vi "Teleop.vi"(10 "Match Info":T2={"Autonomous Elapsed Seconds"=0.0, "TeleOp Elapsed Seconds"=0.0, "Disabled Elapsed Seconds"=0.0, "Visited Autonomous"=FALSE, "Visited TeleOp"=FALSE, "Visited Disabled"=FALSE, "Autonomous Settings"={"Autonomous Style"=enum."Independent", "VI Refnum"=refnum}}, 11 "Call Context":T3) -> ()   [LabVIEW 2014]
doc: "This VI is called for each TeleOp packet received from the DS where the robot is not disabled. It is often used to read from the joysticks and update I/O or to update setpoints for timed control loops. It should complete and return within 20 milliseconds or it may miss DS packets."
uses:
  <vilib>/Rock Robotics/WPI/DriverStation/WPI_DriverStationDerivedRobotMode.ctl
  <vilib>/Rock Robotics/WPI/DriverStation/WPI_DriverStationMatch Info.ctl
  <vilib>/Rock Robotics/WPI/Joystick/WPI_JoystickGetSetRefNum.vi
  Botones Global.vi
  <vilib>/Rock Robotics/Network Tables/SD Write Boolean Array.vi
  <vilib>/Rock Robotics/Network Tables/SD Write Numeric Array.vi
  <vilib>/Rock Robotics/Network Tables/SD Read Boolean.vi
  <vilib>/Rock Robotics/Network Tables/SD Read Number.vi
  Drive Global.vi
  2283_Outputs autonomo.vi
panel:
  in  "Outputs autonomo":T1
  in  "drive":cluster{"Eje 0":dbl, "Eje 1":dbl, "Eje 2":dbl}
  out "Sample Slider 0":dbl(slide) scale=0.0..5.0
  out "Sample Boolean 1":bool
  out "Sample Boolean 0":bool
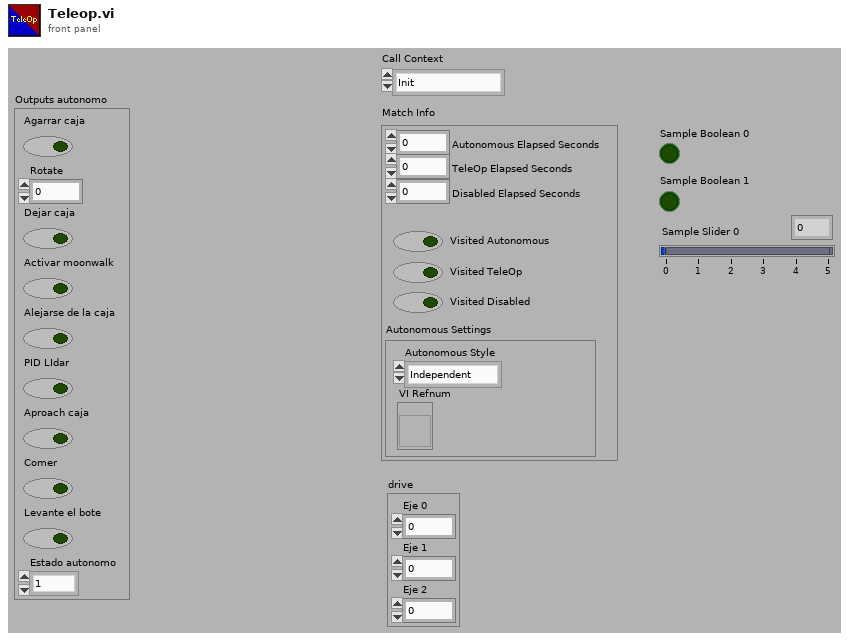
[diagram p1: front panel]
types:
  T1 = cluster{"Agarrar caja":bool, "Rotate":dbl, "Dejar caja":bool, "Activar moonwalk":bool, "Alejarse de la caja":bool, "PID LIdar":bool, "Aproach caja":bool, "Comer":bool, "Levante el bote":bool, "Estado autonomo":enum16{"1", "2", "3", "4", "5", "6", "7", "8", "9", "10", "11", "12"}}
  T2 = typedef "WPI_DriverStationMatch Info.ctl" = cluster{"Autonomous Elapsed Seconds":dbl, "TeleOp Elapsed Seconds":dbl, "Disabled Elapsed Seconds":dbl, "Visited Autonomous":bool, "Visited TeleOp":bool, "Visited Disabled":bool, "Autonomous Settings":cluster{"Autonomous Style":enum16{"Iterative", "Independent"}, "VI Refnum":refnum<vi>}}
  T3 = typedef "WPI_DriverStationDerivedRobotMode.ctl" = enum16{"Init", "Execute", "Stop"}
  T4 = typedef "WPI_JoystickDevRef.ctl" = cluster{"Device":T5}
  T5 = typedef "WPI_JoystickDeviceEnum.ctl" = enum16{"USB 0", "USB 1", "USB 2", "USB 3", "USB 4", "USB 5"}
  T6 = cluster{"Axes[0]":dbl, "Axes[1]":dbl, "Axes[2]":dbl, "Axes[3]":dbl, "Axes[4]":dbl, "Axes[5]":dbl, "Axes[6]":dbl, "Axes[7]":dbl, "Axes[8]":dbl}
  T7 = cluster{"Buttons[0]":bool, "Buttons[1]":bool, "Buttons[2]":bool, "Buttons[3]":bool, "Buttons[4]":bool, "Buttons[5]":bool, "Buttons[6]":bool, "Buttons[7]":bool, "Buttons[8]":bool}
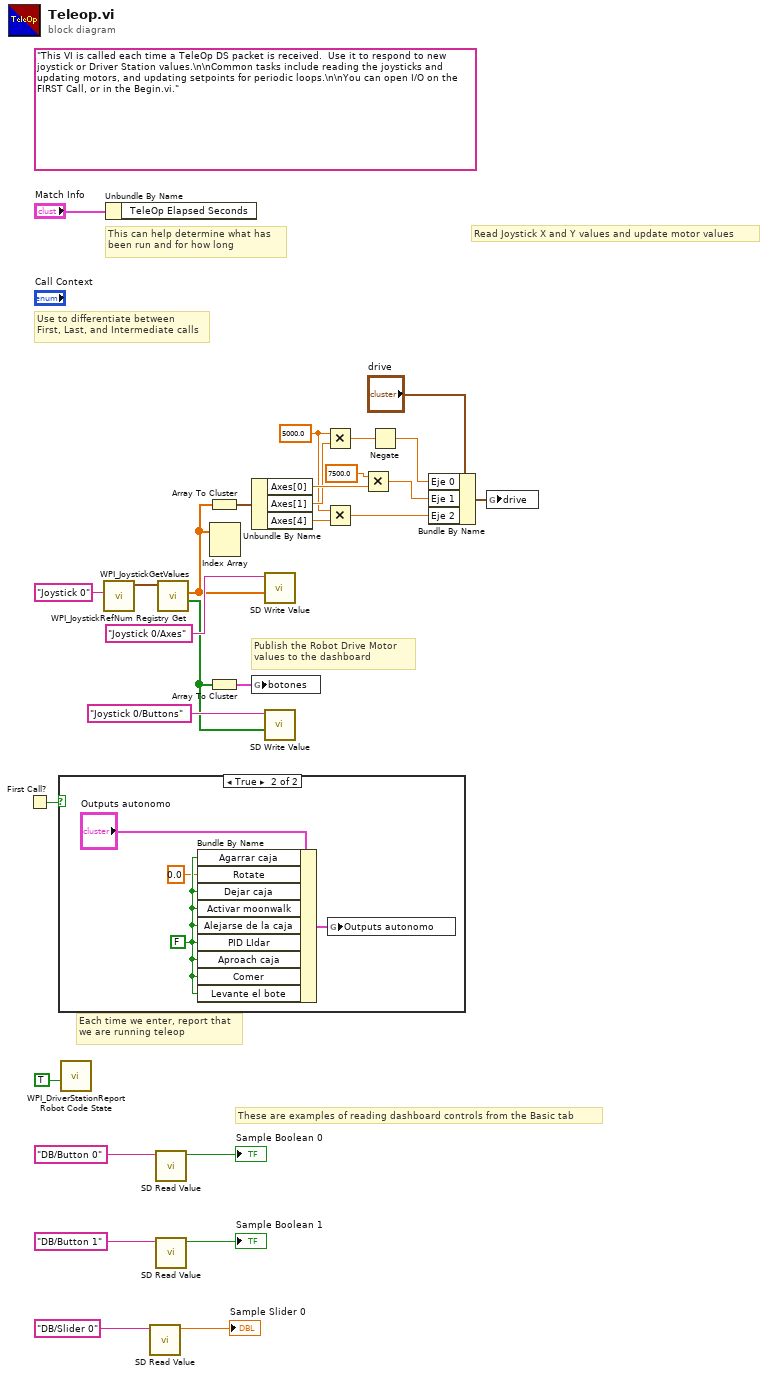
[diagram p0: block diagram]
diagram:
  w6 = 5000.0
  (unwired) "This VI is called each time a TeleOp DS packet is received.  Use it to respond to new joystick or Driver Station values.\n\nCommon tasks include reading the joysticks and updating motors, and updating setpoints for periodic loops.\n\nYou can open I/O on the FIRST Call, or in the Begin.vi."
  # "These are examples of reading dashboard controls from the Basic tab"
  # "Publish the Robot Drive Motor\nvalues to the dashboard"
  # "Each time we enter, report that\nwe are running teleop"
  # "Use to differentiate between\nFirst, Last, and Intermediate calls"
  # "This can help determine what has\nbeen run and for how long"
  # "Read Joystick X and Y values and update motor values"
  n1 = First Call?() -> (First Call?: T/F=w1:bool)
  n2 = case shown="True" w1 {
    frame False {
    }
    frame True {
      w30 = FALSE ("Agarrar caja")
      n3 = Bundle By Name(cluster="Outputs autonomo", "Agarrar caja"=w30, "Rotate"=0.0, "Dejar caja"=w30, "Activar moonwalk"=w30, "Alejarse de la caja"=w30, "PID LIdar"=w30, "Aproach caja"=w30, "Comer"=w30, "Levante el bote"=w30) -> (w32:T1)
      n4 = global write "2283_Outputs autonomo.vi" "Outputs autonomo"(w32) -> ()
    }
  }
  n5 = call <vilib>:"WPI_DriverStationReport Robot Code State.vi"("TeleOp"=TRUE ("Autonomous")) -> ()  [unwired: 10 in, 1 out]
  n6 = call <vilib>:"WPI_JoystickRefNum Registry Get.vi"("refnum name"="Joystick 0") -> ("JoystickDevRef"=w26:T4)  [unwired: 1 in, 9 out]
  n7 = Unbundle By Name("Match Info") -> ()  [unwired: 1 out]
  n8 = call-poly <vilib>:"SD Read Value.vi"("Name"="DB/Slider 0" ("refnum name")) -> ("Numeric"=→"Sample Slider 0":dbl)  [unwired: 8 in, 2 out]
  n9 = call-poly <vilib>:"SD Read Value.vi"("Name"="DB/Button 0" ("refnum name")) -> ("Boolean"=→"Sample Boolean 0":bool)  [unwired: 8 in, 2 out]
  n10 = call-poly <vilib>:"SD Read Value.vi"("Name"="DB/Button 1" ("refnum name")) -> ("Boolean"=→"Sample Boolean 1":bool)  [unwired: 8 in, 2 out]
  n11 = call <vilib>:"WPI_JoystickGetValues.vi"("JoystickDevRef"=w26) -> ("Buttons"=w12:bool[], "Axes"=w16:dbl[])  [unwired: 6 in, 3 out]
  n12 = Array To Cluster(array=w16) -> (cluster=w15:T6)
  n13 = Array To Cluster(array=w12) -> (cluster=w11:T7)
  n14 = Index Array(array=w16) -> ()  [unwired: 2 in, 2 out]
  n15 = Unbundle By Name(w15) -> ("Axes[0]"=w10:dbl, "Axes[1]"=w9:dbl, "Axes[4]"=w7:dbl)
  n16 = global write "Botones Global.vi" "botones"(w11) -> ()
  n17 = call-poly <vilib>:"SD Write Value.vi"("Numeric Array"=w16, "Name"="Joystick 0/Axes") -> ()  [unwired: 8 in, 2 out]
  n18 = call-poly <vilib>:"SD Write Value.vi"("Boolean Array"=w12, "Name"="Joystick 0/Buttons") -> ()  [unwired: 8 in, 2 out]
  n19 = Multiply(x=w6, y=w9) -> (x*y=w4:dbl)
  n20 = Multiply(x=w6, y=w7) -> (x*y=w8:dbl)
  n21 = Multiply(x=7500.0, y=w10) -> (x*y=w5:dbl)
  n22 = Negate(x=w4) -> (-x=w3:dbl)
  n23 = Bundle By Name(cluster="drive", "Eje 0"=w3, "Eje 1"=w5, "Eje 2"=w8) -> (w13:cluster{"Eje 0":dbl, "Eje 1":dbl, "Eje 2":dbl})
  n24 = global write "Drive Global.vi" "drive"(w13) -> ()
